vi "Get Message Transport Notifier.vi"(8 "error in (no error)":errorcluster, 11 "Message Transport Notifier in":refnum<class "Message Transport Notifier.lvclass">) -> (0 "error out":errorcluster, 3 "Notifier":refnum<notifier>)   [LabVIEW 2016, in "Stream Mediator.lvlib" / "Message Transport Notifier.lvclass"]
doc: "--\nCopyright © 2017 Composed SystemsI All rights reserved.\n\nAuthor: Jon McBee <jon.mcbee@composed.io>\n\nThis library is provided \"AS IS\" ,WITHOUT WARRANTIES OR\nCONDITIONS OF ANY KIND, either express or implied.\n\nComposed Systems -- composed.io\n\nStream 0.0.1.1\nJon McBee - Composed Systems\nCopyright (c) 2017, Composed Systems"
uses:
  <userlib>/Composed Systems/Stream/Mediator/Classes/Message Transport Notifier/Message Transport Notifier.lvclass
  <userlib>/Composed Systems/Stream/Mediator/Classes/Message Interface/Message Interface.lvclass
  <userlib>/Composed Systems/Stream/Mediator/Classes/Message Transport Notifier/Message Transport Notifier.lvclass/Message Transport Notifier.ctl
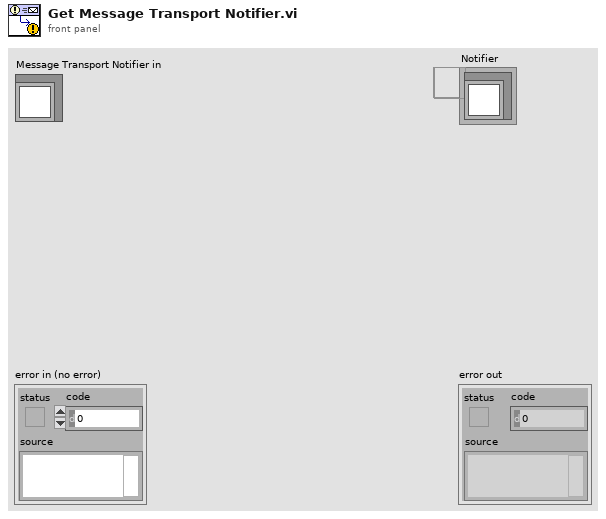
[diagram p1: front panel]
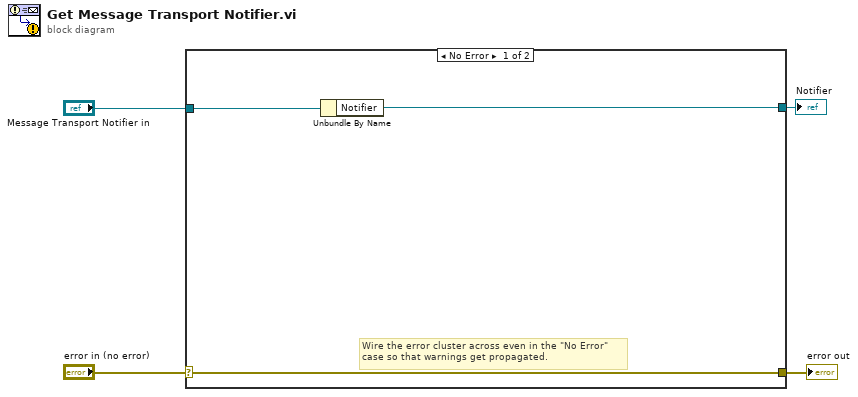
[diagram p0: block diagram]
diagram:
  n1 = case shown="No Error" "error in (no error)" {
    selector: "error in (no error)" -> [w7 w8]
    tunnel: [w7 w8] -> w3
    tunnel: "Message Transport Notifier in" -> [w6 _]
    tunnel: [w5 _] -> w1
    frame No Error {
      # "Wire the error cluster across even in the \"No Error\"\ncase so that warnings get propagated."
      n2 = Unbundle By Name(w6) -> ("Notifier"=w5:refnum<notifier>)
    }
    frame Error {
    }
  }
  "error out" <- w3
  "Notifier" <- w1
